vi "External Transition.vi"(8 "error in (no error)":errorcluster, 9 "Timeout Period in ms (-1, never)":i32=-1, 10 "Target State":refnum<class "_State Machine Actor.lvclass">, 11 "State Machine Actor in":refnum<class "State Machine Actor.lvclass">) -> (0 "error out":errorcluster, 3 "_State Machine Actor out":refnum<class "_State Machine Actor.lvclass">)   [LabVIEW 2024, in "State Machine Actor.lvlib" / "State Machine Actor.lvclass"]
uses:
  State Machine Actor.lvclass
  State Machine Actor.lvclass/State Machine Actor.ctl
  _State Machine Actor/_State Machine Actor/_State Machine Actor.lvclass
  C:/Users/uspoaotto/OneDrive - Oregon Tool/Desktop/working copies/stateMachineActor/src/_State Machine Actor/_State Machine Actor/_State Machine Actor.lvclass
  C:/Program Files (x86)/National Instruments/LabVIEW 2024/vi.lib/ActorFramework/Actor/Actor.lvclass
  C:/Users/uspoaotto/OneDrive - Oregon Tool/Desktop/working copies/stateMachineActor/src/State Machine Actor/State Machine Actor/State Machine Actor.lvclass
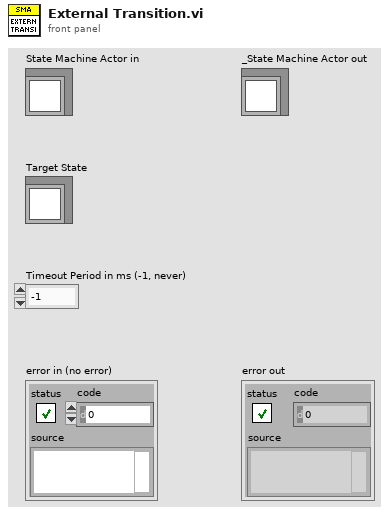
[diagram p1: front panel]
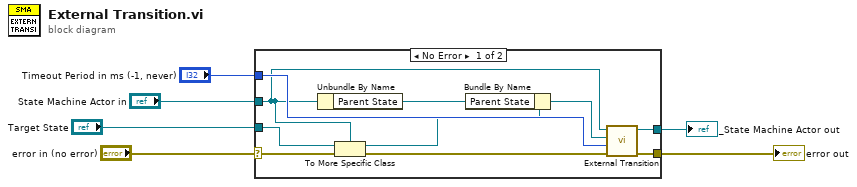
[diagram p0: block diagram]
diagram:
  n1 = case shown="No Error" "error in (no error)" {
    selector: "error in (no error)" -> [w7 w17]
    tunnel: [w16 w17] -> w6
    tunnel: [w15 w18] -> w5
    tunnel: "Timeout Period in ms (-1, never)" -> [w14 _]
    tunnel: "State Machine Actor in" -> [w13 w18]
    tunnel: "Target State" -> [w12 _]
    frame No Error {
      n2 = Unbundle By Name(w13) -> ("Parent State"=w9:refnum<class "_State Machine Actor.lvclass">)
      n3 = To More Specific Class(target class=w13, reference=w12, error in=w7) -> (specific class reference=w10:refnum<class "State Machine Actor.lvclass">, error out=w11:errorcluster)
      n4 = Bundle By Name(cluster=w10, "Parent State"=w9) -> (w8:refnum<class "State Machine Actor.lvclass">)
      n5 = call-parent "External Transition.vi"("error in (no error)"=w11, "Timeout Period in ms (-1, never)"=w14, "Target State"=w8, "_State Machine Actor in"=w13) -> ("error out"=w16:errorcluster, "_State Machine Actor out"=w15:refnum<class "_State Machine Actor.lvclass">)  [unwired: 6 in]
    }
    frame Error {
    }
  }
  "error out" <- w6
  "_State Machine Actor out" <- w5
